vi "TCP serial camera encode.vi"(9 "Camera Controls":T1) -> (1 "camera commands":string[](array[string]))   [LabVIEW 2021]
uses:
  Controls/Host - GUI Data Cluster.ctl
  Analog Output/Controls/AO JSON Data Cluster.ctl
  Analog Output/Controls/AO Interface Data Cluster.ctl
  Analog Output/Controls/AO Channel Configuration Cluster.ctl
  Analog Output/Controls/AO Timing Cluster.ctl
  Digital Output/Controls/DIO Configuration cluster.ctl
  Digital Output/Controls/DIO Interface Data.ctl
  Digital Output/SubVIs/Digital Dynamic Cluster.ctl
  Async JSON Cluster.ctl
  Async Interface Data Cluster.ctl
  Async Serial/Controls/Async Serial Configuration Cluster.ctl
  Async Serial/Controls/Async Frame Info Cluster.ctl
  Async Serial/Controls/Async Message Info Cluster.ctl
  Controls/Host Data Cluster.ctl
  Main Engine/Controls/Main Engine CPU Info.ctl
panel:
  out "Array 1":u8[](array[numeric])
  in  "Numeric":u32
  out "Array 2":u8[](array[numeric])
  in  "Data Cluster":T2={"VI References"=[], "Addresses"=[], "Pilot"=FALSE, "DO Data"=[], "Access Restricted?"=FALSE, "Pilot Control References"=[], "CoPilot Control References"=[], "cRIO Config"=[], "datalog Q"=refnum, "PS_P"={"AI"=[], "DI"=[], "DO"=[], "Serial"=[], "CPU"={"Total Load"=[], "Interrupt Load"=[], "Total Physical"=0.0, "Free Physical"=0.0, "Primary Disk Capacity"=0.0, "Primary Disk Free"=0.0}, "Stop"=FALSE, "DO Channel"=[]}, "PS_S"={"AI"=[], "DI"=[], "DO"=[], "Serial"=[], "CPU"={"Total Load"=[], "Interrupt Load"=[], "Total Physical"=0.0, "Free Physical"=0.0, "Primary Disk Capacity"=0.0, "Primary Disk Free"=0.0}, "Stop"=FALSE, "DO Channel"=[]}, "IDE_P"={"AI"=[], "DI"=[], "DO"=[], "Serial"=[], "CPU"={"Total Load"=[], "Interrupt Load"=[], "Total Physical"=0.0, "Free Physical"=0.0, "Primary Disk Capacity"=0.0, "Primary Disk Free"=0.0}, "Stop"=FALSE, "DO Channel"=[]}, "IDE_S"={"AI"=[], "DI"=[], "DO"=[], "Serial"=[], "CPU"={"Total Load"=[], "Interrupt Load"=[], "Total Physical"=0.0, "Free Physical"=0.0, "Primary Disk Capacity"=0.0, "Primary Disk Free"=0.0}, "Stop"=FALSE, "DO Channel"=[]}, "PDE_P"={"AI"=[], "DI"=[], "DO"=[], "Serial"=[], "CPU"={"Total Load"=[], "Interrupt Load"=[], "Total Physical"=0.0, "Free Physical"=0.0, "Primary Disk Capacity"=0.0, "Primary Disk Free"=0.0}, "Stop"=FALSE, "DO Channel"=[]}, "PDE_S"={"AI"=[], "DI"=[], "DO"=[], "Serial"=[], "CPU"={"Total Load"=[], "Interrupt Load"=[], "Total Physical"=0.0, "Free Physical"=0.0, "Primary Disk Capacity"=0.0, "Primary Disk Free"=0.0}, "Stop"=FALSE, "DO Channel"=[]}, "GUI References"={"Control Names"=[], "Control References"=[]}, "GUI Data"=[], "TCP - Serial"=[], "TCP-Serial Q"=refnum, "TCP Serial Ref"=[], "Data Sets"=[], "Last Data"=[], "Alarm Data"=[], "DI Data"=[], "Ack Data"=[], "Buzzer Data"=[], "Pilot DO"=[], "Co-Pilot DO"=[], "System Down?"=FALSE, "Log Data"=[], "Update Array"=[], "MCC Data Log"=[], "MCC Data Not"=refnum, "Thruster control"=[refnum, refnum, refnum, refnum, refnum, refnum, refnum, refnum, refnum], "waga notifier out"=refnum, "Wago  log"=[], "Thruster Cont"=[0.0, 0.0, 0.0, 0.0, 0.0, 0.0, 0.0, 0.0, 0.0], "Cam Cont"=[FALSE, FALSE, FALSE, FALSE, FALSE, TRUE], "PDE_P TH Cont"={"COM 10"=0.0, "COM 11"=0.0, "COM 12"=0.0, "COM 13"=0.0}, "PDE_S TH Cont"={"COM 10"=0.0, "COM 11"=0.0, "COM 12"=0.0, "COM 13"=0.0}} {"cRIO Config"."AI"."Interface Data"."Timing"."sample mode" items=["Finite Samples"=10178, "Continuous Samples"=10123, "Hardware Timed Single Point"=12522]; "cRIO Config"."Async"."Interface Data"."Data"."Minor Frame Count" min=5 max=8 step=1}
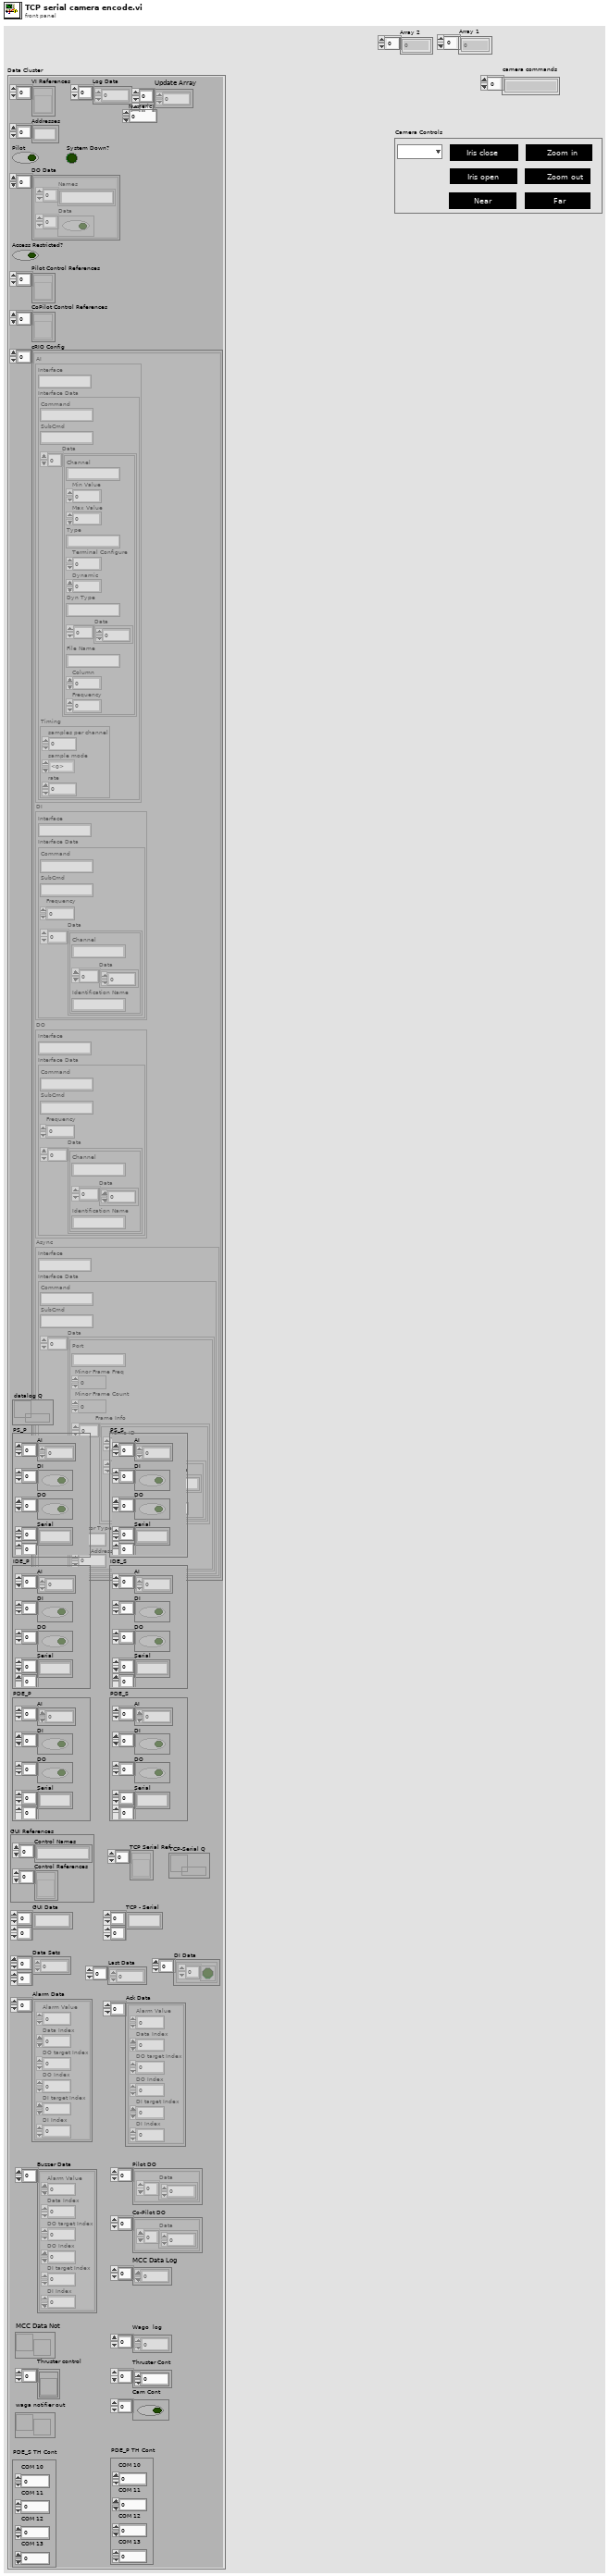
[diagram p1: front panel]
types:
  T1 = cluster{"Enum - Menu":enum16{"", "Camera 2", "Camera 1"}, "ZOOM IN":bool, "ZOOM OUT":bool, "IRIS OPEN":bool, "IRIS CLOSE":bool, "ZOOM OUT 2":bool, "IRIS CLOSE 2":bool}
  T2 = typedef "Host - GUI Data Cluster.ctl" = cluster{"VI References":refnum<vi>[], "Addresses":string[], "Pilot":bool, "DO Data":cluster{"Names":string[], "Data":bool[]}[], "Access Restricted?":bool, "Pilot Control References":refnum<vi>[], "CoPilot Control References":refnum<vi>[], "cRIO Config":cluster{"AI":T3, "DI":T7, "DO":T7, "Async":T10}[], "datalog Q":refnum<queue>, "PS_P":T15, "PS_S":T15, "IDE_P":T15, "IDE_S":T15, "PDE_P":T15, "PDE_S":T15, "GUI References":cluster{"Control Names":string[], "Control References":refnum<vi>[]}, "GUI Data":string[][], "TCP - Serial":string[][], "TCP-Serial Q":refnum<queue>, "TCP Serial Ref":refnum<vi>[], "Data Sets":dbl[][], "Last Data":dbl[], "Alarm Data":cluster{"Alarm Value":dbl, "Data Index":i32, "DO target Index":i32, "DO Index":i32, "DI target Index":i32, "DI Index":i32}[], "DI Data":cluster{bool[]}[], "Ack Data":cluster{"Alarm Value":dbl, "Data Index":i32, "DO target Index":i32, "DO Index":i32, "DI target Index":i32, "DI Index":i32}[], "Buzzer Data":cluster{"Alarm Value":dbl, "Data Index":i32, "DO target Index":i32, "DO Index":i32, "DI target Index":i32, "DI Index":i32}[], "Pilot DO":cluster{"Data":i32[]}[], "Co-Pilot DO":cluster{"Data":i32[]}[], "System Down?":bool, "Log Data":dbl[], "Update Array":i32[][], "MCC Data Log":dbl[], "MCC Data Not":refnum<notifier>, "Thruster control":refnum<vi>[], "waga notifier out":refnum<notifier>, "Wago  log":sgl[], "Thruster Cont":dbl[], "Cam Cont":bool[], "PDE_P TH Cont":cluster{"COM 10":dbl, "COM 11":dbl, "COM 12":dbl, "COM 13":dbl}, "PDE_S TH Cont":cluster{"COM 10":dbl, "COM 11":dbl, "COM 12":dbl, "COM 13":dbl}}
  T3 = typedef "AO JSON Data Cluster.ctl" = cluster{"Interface":string, "Interface Data":T4}
  T4 = typedef "AO Interface Data Cluster.ctl" = cluster{"Command":string, "SubCmd":string, "Data":T5[], "Timing":T6}
  T5 = typedef "AO Channel Configuration Cluster.ctl" = cluster{"Channel":string, "Min Value":dbl, "Max Value":dbl, "Type":string, "Terminal Configure":u16, "Dynamic":u8, "Dyn Type":string, "Data":dbl[], "File Name":string, "Column":i32, "Frequency":dbl}
  T6 = typedef "AO Timing Cluster.ctl" = cluster{"samples per channel":i32, "sample mode":i32, "rate":dbl}
  T7 = typedef "DIO Configuration cluster.ctl" = cluster{"Interface":string, "Interface Data":T8}
  T8 = typedef "DIO Interface Data.ctl" = cluster{"Command":string, "SubCmd":string, "Frequency":u16, "Data":T9[]}
  T9 = typedef "Digital Dynamic Cluster.ctl" = cluster{"Channel":string, "Data":u8[], "Identification Name":string}
  T10 = typedef "Async JSON Cluster.ctl" = cluster{"Interface":string, "Interface Data":T11}
  T11 = typedef "Async Interface Data Cluster.ctl" = cluster{"Command":string, "SubCmd":string, "Data":T12[]}
  T12 = typedef "Async Serial Configuration Cluster.ctl" = cluster{"Port":string, "Minor Frame Freq":u16, "Minor Frame Count":u16, "Frame Info":T13[], "Sensor Type":u16, "OIM Address":u16}
  T13 = typedef "Async Frame Info Cluster.ctl" = cluster{"Frame ID":u16, "Message Info":T14[]}
  T14 = typedef "Async Message Info Cluster.ctl" = cluster{"Message":u8[], "Message Name":string}
  T15 = typedef "Host Data Cluster.ctl" = cluster{"AI":dbl[], "DI":bool[], "DO":bool[], "Serial":string[][], "CPU":T16, "Stop":bool, "DO Channel":string[]}
  T16 = typedef "Main Engine CPU Info.ctl" = cluster{"Total Load":u32[], "Interrupt Load":u32[], "Total Physical":dbl, "Free Physical":dbl, "Primary Disk Capacity":dbl, "Primary Disk Free":dbl}
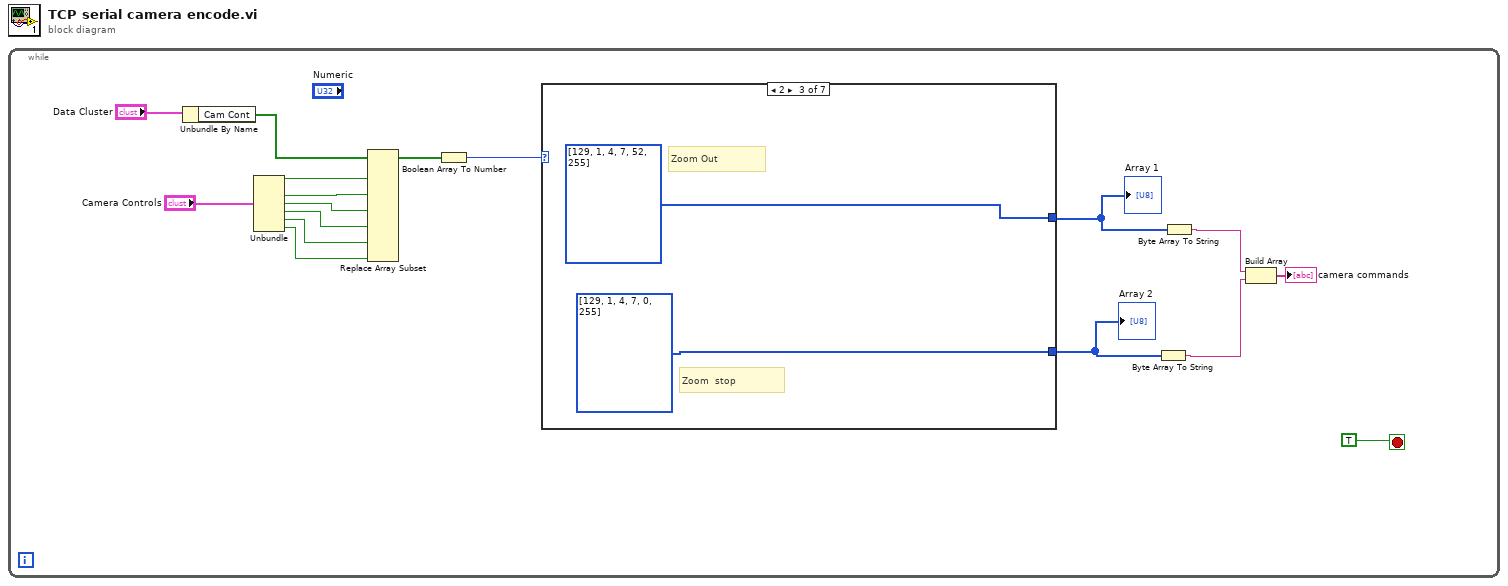
[diagram p0: block diagram]
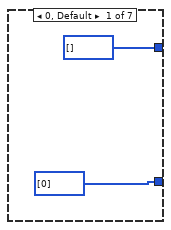
[diagram p2: hidden frame]
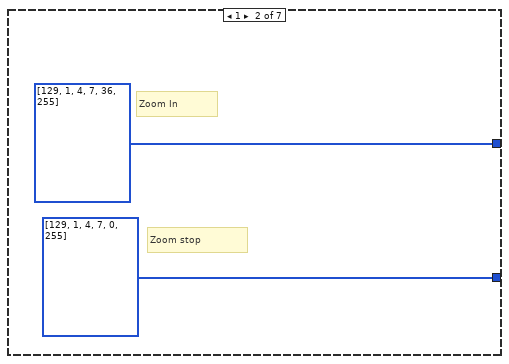
[diagram p3: hidden frame]
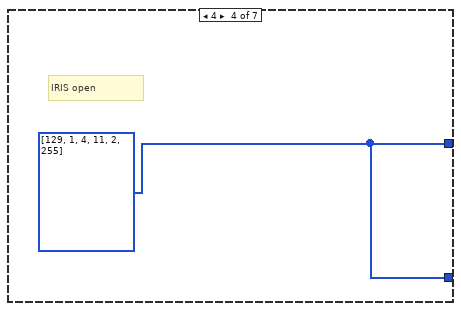
[diagram p4: hidden frame]
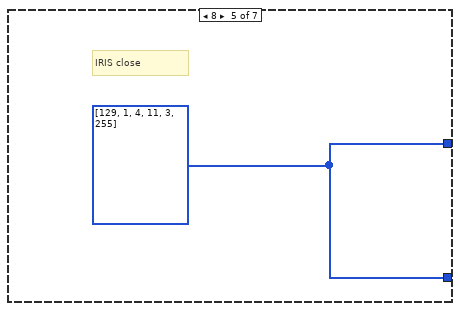
[diagram p5: hidden frame]
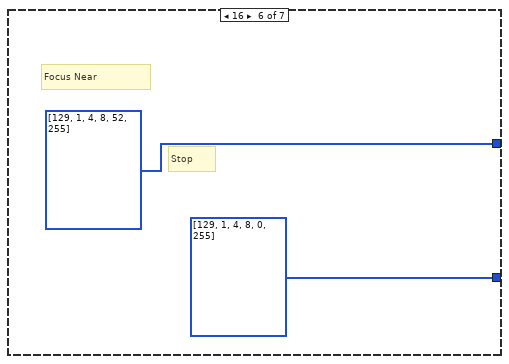
[diagram p6: hidden frame]
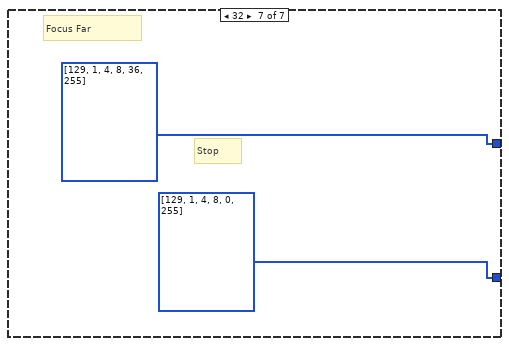
[diagram p7: hidden frame]
diagram:
  n1 = while {
    stop <- TRUE stop-if-true
    n2 = Unbundle By Name("Data Cluster") -> ("Cam Cont"=w15:bool[])
    n3 = Unbundle("Camera Controls") -> ("ZOOM IN"=w7:bool, "ZOOM OUT"=w8:bool, "IRIS OPEN"=w9:bool, "IRIS CLOSE"=w10:bool, "ZOOM OUT 2"=w11:bool, "IRIS CLOSE 2"=w12:bool)  [unwired: 1 out]
    n4 = Replace Array Subset(array=w15, new element #1=w7, new element #2=w8, new element #3=w9, new element #4=w10, new element #5=w11, new element #6=w12) -> (w13:bool[])  [unwired: 6 in]
    n5 = Boolean Array To Number(Boolean array=w13) -> (number=w5:u32)
    n6 = case shown="2" w5 {
      tunnel: [u8[] [] u8[] [129, 1, 4, 7, 36, 255] u8[] [129, 1, 4, 7, 52, 255] w24 w25 u8[] [129, 1, 4, 8, 52, 255] u8[] [129, 1, 4, 8, 36, 255]] -> w17
      tunnel: [u8[] [0] u8[] [129, 1, 4, 7, 0, 255] u8[] [129, 1, 4, 7, 0, 255] w24 w25 u8[] [129, 1, 4, 8, 0, 255] u8[] [129, 1, 4, 8, 0, 255]] -> w16
      frame 0, Default {
      }
      frame 1 {
        # "Zoom stop"
        # "Zoom In"
      }
      frame 2 {
        # "Zoom  stop"
        # "Zoom Out"
      }
      frame 4 {
        w24 = u8[] [129, 1, 4, 11, 2, 255]
        # "IRIS open"
      }
      frame 8 {
        w25 = u8[] [129, 1, 4, 11, 3, 255]
        # "IRIS close"
      }
      frame 16 {
        # "Stop"
        # "Focus Near"
      }
      frame 32 {
        # "Stop"
        # "Focus Far"
      }
    }
    "Array 1" <- w17
    "Array 2" <- w16
    n7 = Byte Array To String(unsigned byte array=w16) -> (string=w3:string)
    n8 = Byte Array To String(unsigned byte array=w17) -> (string=w4:string)
    n9 = Build Array(w4, w3) -> (→"camera commands":string[])
  }
